vi "Feather Plot.vi"() -> ()   [LabVIEW 2013]
doc: "This VI shows how to use the 2D Feather Plot."
uses:
  <vilib>/Math Plots/2D Math Plots/2D Feather/2D Feather XCtrl/2D Feather.xctl
  <vilib>/Math Plots/2D Math Plots/2D Compass/2D Compass XCtrl/2D Compass.xctl
  <vilib>/Math Plots/2D Math Plots/2D Compass/2D Compass Datatype/Public/Plot Helper (Complex).vi
  <vilib>/Math Plots/2D Math Plots/2D Feather/2D Feather Datatype/Public/Plot Helper (Complex).vi
  <vilib>/Math Plots/2D Math Plots/2D Feather/2D Feather Datatype/2D Feather Datatype.lvclass
  <vilib>/Math Plots/2D Math Plots/2D Compass/2D Compass Datatype/2D Compass Datatype.lvclass
panel:
  out "2D Compass":refnum<class "2D Plot Datatype.lvclass">[](xcontrol)
  in  "Dial":dbl(knob)
  in  "r":dbl(slide) scale=-10.0..10.0
  in  "stop":bool
  out "Direction":dbl
  out "Velocity":dbl
  out "Acceleration":dbl
  out "Feather Plot":refnum<class "2D Plot Datatype.lvclass">[](xcontrol)
  # "Overview: Demonstrates the Feather Plot indicator.\nInstructions:\nRun the VI."
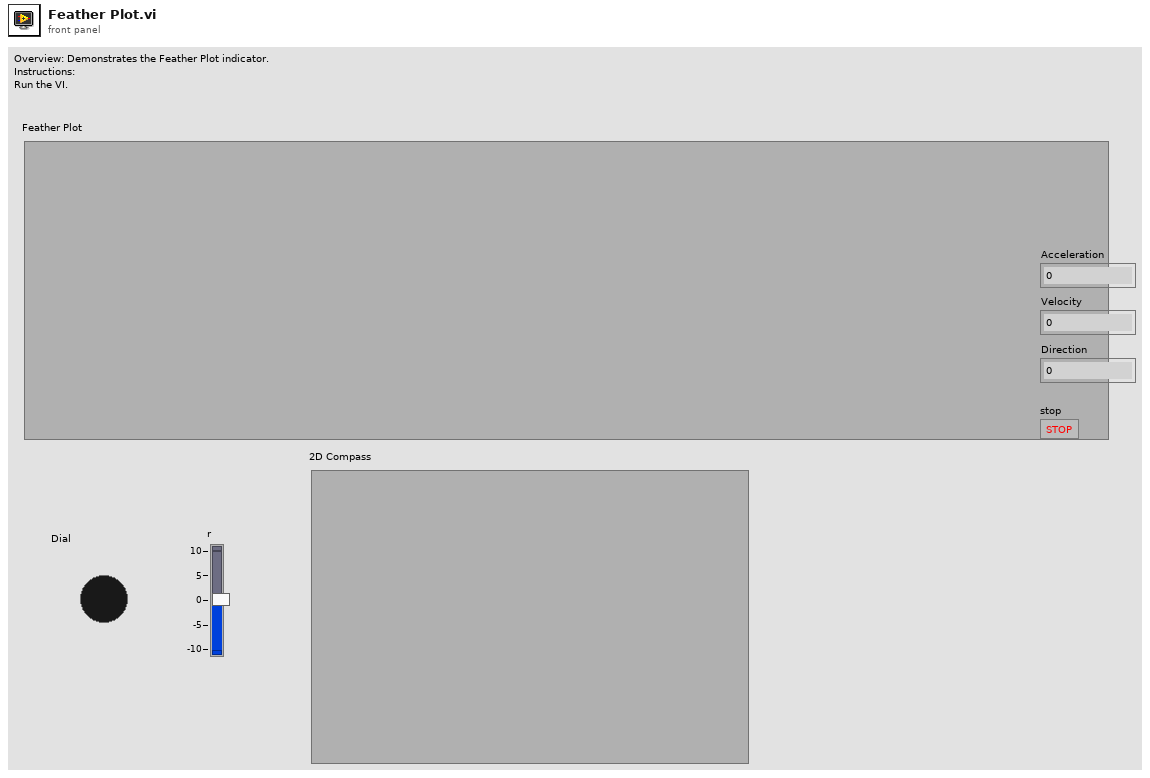
[diagram p1: front panel]
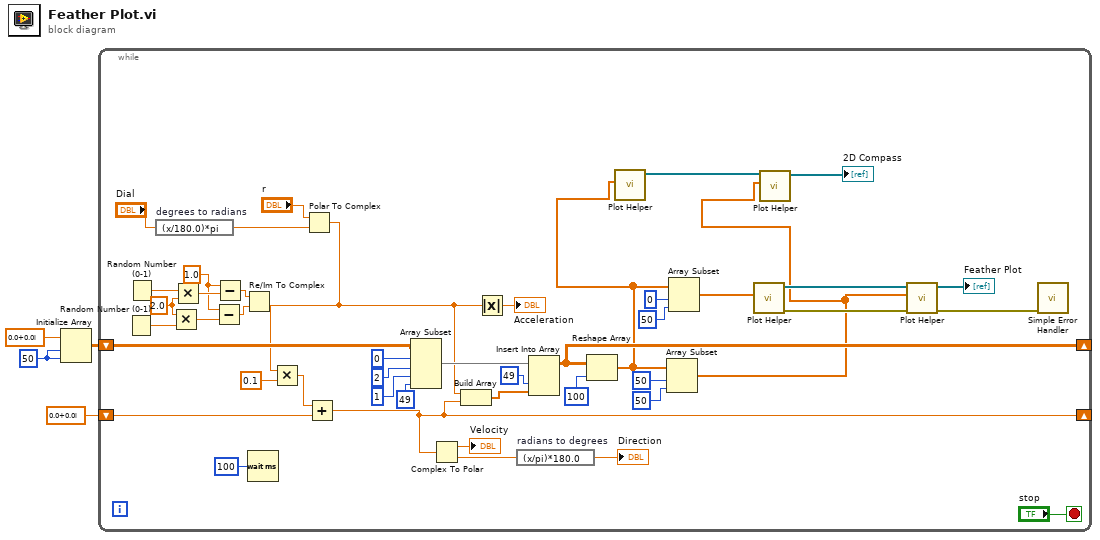
[diagram p0: block diagram]
diagram:
  w1 = 50 ("dimension size")
  n1 = Initialize Array(cdb 0.0+0.0i ("x"), w1, w1) -> (w3:cdb[][])
  n2 = while {
    shift-right: [w31] -> _
    shift-left: cdb 0.0+0.0i ("x") -> [w43]
    shift-right: [w30] -> _
    shift-left: w3 -> [w38]
    stop <- "stop" stop-if-true
    w14 = 2.0 ("y")
    w17 = 1.0 ("x")
    n3 = Random Number (0-1)() -> (number: 0 to 1=w20:dbl)
    n4 = Random Number (0-1)() -> (number: 0 to 1=w21:dbl)
    n5 = expression code="(x/180.0)*pi" "degrees to radians"("Dial") -> (w11:dbl)
    n6 = Multiply(x=w14, y=w20) -> (x*y=w18:dbl)
    n7 = Multiply(x=w21, y=w14) -> (x*y=w19:dbl)
    n8 = Subtract(x=w17, y=w18) -> (x-y=w15:dbl)
    n9 = Subtract(x=w17, y=w19) -> (x-y=w16:dbl)
    n10 = Re/Im To Complex(1:w15, 2:w16) -> ()  [unwired: 1 out]
    n11 = Wait (ms)(milliseconds to wait=u32 100) -> ()  [unwired: 1 out]
    n12 = Polar To Complex(1:w11, 2:"r") -> (0:w12:cdb)
    n13 = Multiply(x=w12, y=0.1) -> (x*y=w45:cdb)
    n14 = Add(x=w45, y=w43) -> (x+y=w31:cdb)
    n15 = Array Subset(array=w38, index (row)=0 ("index"), length (row)=2 ("length"), index (col)=1 ("index"), length (col)=49 ("length")) -> (w37:cdb[][])
    n16 = Complex To Polar(r * e^(i*theta)=w31) -> (r=→"Velocity":dbl, theta=w47:dbl)
    n17 = Build Array(w12, w31) -> (w32:cdb[])
    n18 = Absolute Value(x=w12) -> (abs(x)=→"Acceleration":dbl)
    n19 = expression code="(x/pi)*180.0" "radians to degrees"(w47) -> (→"Direction":dbl)
    n20 = Insert Into Array(array=w37, index (col)=49 ("index (row)"), new element=w32) -> (w30:cdb[][])  [unwired: 1 in]
    n21 = Reshape Array(w30, 100 ("dimension size")) -> (w5:cdb[])
    n22 = call-poly <vilib>:"Plot Helper.vi"("z vector"=w5) -> ("2D Plot Class Obj Array out"=w7:refnum<class "2D Plot Datatype.lvclass">[])  [unwired: 2 in, 8 out]
    n23 = Array Subset(array=w5, index=50, length=50) -> (w6:cdb[])
    n24 = Array Subset(array=w5, index=0, length=50) -> (w9:cdb[])
    n25 = call-poly <vilib>:"Plot Helper.vi"("z vector"=w9) -> ("error out"=w23:errorcluster, "2D Plot Class Obj Array out"=w28:refnum<class "2D Plot Datatype.lvclass">[])  [unwired: 2 in, 7 out]
    n26 = call-poly <vilib>:"Plot Helper.vi"("z vector"=w6, "2D Plot Class Obj Array in"=w7) -> ("2D Plot Class Obj Array out"=→"2D Compass":refnum<class "2D Plot Datatype.lvclass">[])  [unwired: 1 in, 8 out]
    n27 = call-poly <vilib>:"Plot Helper.vi"("error in (no error)"=w23, "z vector"=w6, "2D Plot Class Obj Array in"=w28) -> ("error out"=w40:errorcluster, "2D Plot Class Obj Array out"=→"Feather Plot":refnum<class "2D Plot Datatype.lvclass">[])  [unwired: 7 out]
    n28 = call <vilib>:"Simple Error Handler.vi"("error in (no error)"=w40) -> ()  [unwired: 4 in, 5 out]
  }
